vi "simpleclient.vi"   [LabVIEW 2017]
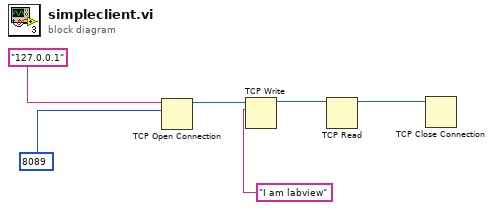
[diagram p0: block diagram]
diagram:
  n1 = TCP Open Connection(address="127.0.0.1", remote port or service name=8089) -> (connection ID=w4:refnum<k5>)  [unwired: 3 in, 1 out]
  n2 = TCP Write(connection ID=w4, data in="I am labview") -> (connection ID out=w3:refnum<k5>)  [unwired: 2 in, 2 out]
  n3 = TCP Read(connection ID=w3) -> (connection ID out=w2:refnum<k5>)  [unwired: 4 in, 2 out]
  n4 = TCP Close Connection(connection ID=w2) -> ()  [unwired: 2 in, 2 out]
